vi "log viewer.vi"() -> ()   [LabVIEW 2010]
uses:
  <vilib>/robotics/Controls/Compass Indicator/Compass Indicator.xctl
  <vilib>/robotics/Controls/Attitude Indicator/Attitude Indicator.xctl
panel:
  in  "play/pause":bool
  in  "stop":bool
  out "Attitude Indicator":cluster{"Roll":dbl, "Pitch":dbl}(xcontrol)
  out "Compass Indicator":dbl(xcontrol)
  out "Buoy Video":T1(plugin-control)
  out "GPS Data":T2 {"Easting" format="%#.10f"; "Northing" format="%#.10f"}
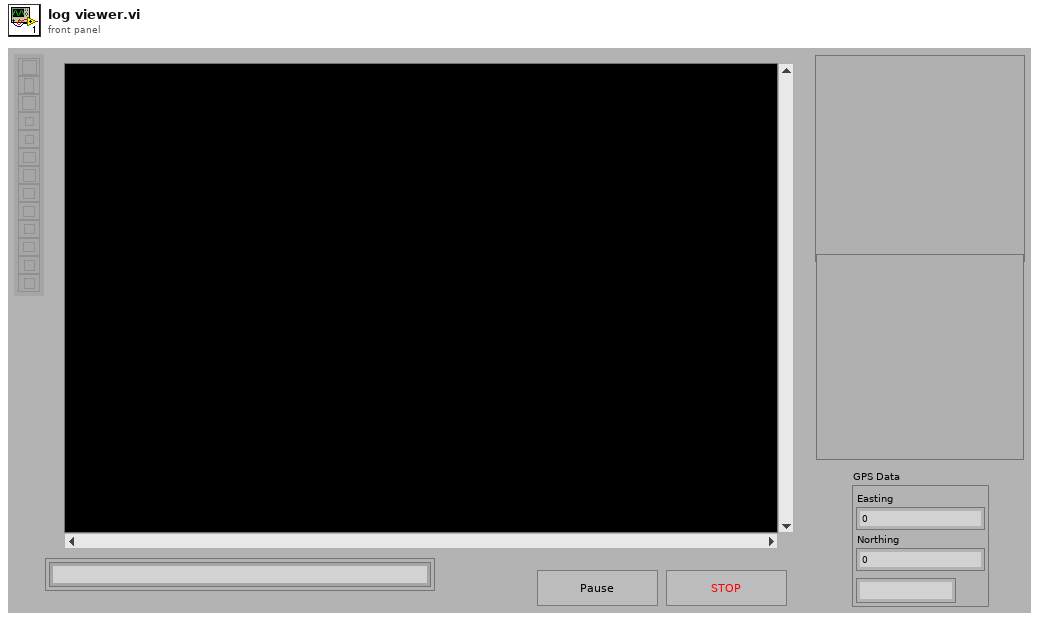
[diagram p1: front panel]
types:
  T1 = typedef "IMAQ Image.ctl" = refnum<image>
  T2 = cluster{"Easting":dbl, "Northing":dbl, "Status":string}
  T3 = typedef "Image Type" = u32
  T4 = typedef "AviRefnum.ctl" = refnum<k1>
  T5 = cluster{"GPS Data":cluster{"Easting":dbl, "Northing":dbl, "Status":string}, "Compass Data":cluster{"Heading (deg)":dbl, "Pitch (deg)":dbl, "Roll (deg)":dbl}}
  T6 = cluster{"Heading (deg)":dbl, "Pitch (deg)":dbl, "Roll (deg)":dbl}
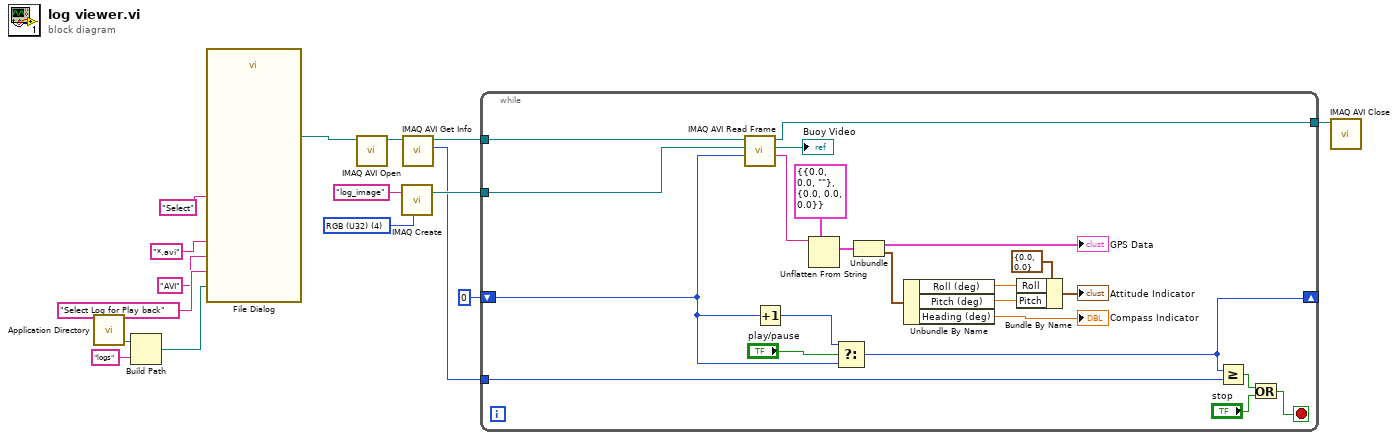
[diagram p0: block diagram]
diagram:
  w6 = T3 4 items=["Grayscale (U8)", "Grayscale (I16)", "Grayscale (SGL)", "Complex (CSG)", "RGB (U32)", "HSL (U32)", "RGB (U64)", "Grayscale (U16)"] ("Image Type")
  n1 = call <vilib>:"Application Directory.vi"() -> ("Application Directory"=w14:path)
  n2 = Build Path(base path=w14, name or relative path="logs") -> (appended path=w15:path)
  n3 = call "File Dialog"("start path"=w15, "prompt"="Select Log for Play back", "button label"="Select", "pattern (all files)"="*.avi", "pattern label"="AVI") -> ("selected path"=w16:path)  [unwired: 7 in, 3 out]
  n4 = call "IMAQ AVI Open"("AVI Path"=w16) -> ("Avi Refnum"=w2:T4)  [unwired: 9 in, 1 out]
  n5 = call "IMAQ Create"("Image Name"="log_image", "Image Type"=w6) -> ("New Image"=w8:T1)  [unwired: 3 in, 1 out]
  n6 = call "IMAQ AVI Get Info"("Avi Refnum"=w2) -> ("Number of Frames"=w1:u32, "Avi Refnum (duplicate)"=w3:T4)  [unwired: 6 in, 3 out]
  n7 = while {
    tunnel: w3 -> [w27]
    tunnel: w8 -> [w26]
    tunnel: [w25] -> w5
    shift-right: [w21] -> _
    shift-left: u32 0 -> [w22]
    tunnel: w1 -> [w20]
    stop <- w17 stop-if-true
    n8 = call "IMAQ AVI Read Frame"("Frame Number"=w22, "Image"=w26, "Avi Refnum"=w27) -> ("Data Out"=w29:string, "Image Out"=→"Buoy Video":T1, "Avi Refnum (duplicate)"=w25:T4)  [unwired: 5 in, 1 out]
    n9 = Increment(x=w22) -> (x+1=w23:u32)
    n10 = Unflatten From String(type=T5 {"GPS Data"={"Easting"=0.0, "Northing"=0.0, "Status"=""}, "Compass Data"={"Heading (deg)"=0.0, "Pitch (deg)"=0.0, "Roll (deg)"=0.0}}, binary string=w29) -> (value=w37:T5)  [unwired: 3 in, 2 out]
    n11 = Select(t=w23, s="play/pause", f=w22) -> (s? t:f=w21:u32)
    n12 = Unbundle(w37) -> ("GPS Data"=→"GPS Data":T2, "Compass Data"=w30:T6)
    n13 = Unbundle By Name(w30) -> ("Roll (deg)"=w34:dbl, "Pitch (deg)"=w35:dbl, "Heading (deg)"=→"Compass Indicator":dbl)
    n14 = Bundle By Name(cluster=cluster{"Roll":dbl, "Pitch":dbl} {"Roll"=0.0, "Pitch"=0.0} ("Attitude Indicator"), "Roll"=w34, "Pitch"=w35) -> (→"Attitude Indicator":cluster{"Roll":dbl, "Pitch":dbl})
    n15 = Greater Or Equal?(x=w21, y=w20) -> (x >= y?=w19:bool)
    n16 = Or(x=w19, y="stop") -> (x .or. y?=w17:bool)
  }
  n17 = call "IMAQ AVI Close"("Avi Refnum"=w5) -> ()  [unwired: 10 in, 1 out]
